vi "Global_scelta_linea.vi"() -> ()   [LabVIEW 2019]
panel:
  in  "Linea selezionata":i16
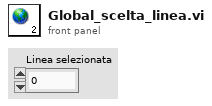
[diagram p1: front panel]
diagram:
